vi "Load DC Pins.vi"(8 "error in (no error)":errorcluster, 11 "DCPower in":refnum<class "DCPower.lvclass">) -> (0 "error out":errorcluster, 3 "DCPower out":refnum<class "DCPower.lvclass">)   [LabVIEW 2018, in "DCPower.lvlib" / "DCPower.lvclass"]
uses:
  DCPower.lvclass
  C:/Sequence Automation/Plugins/Measurement Interface.lvlibp/Measurement Interface.lvclass
  DCPower.lvclass/DCPower.ctl
  Write DC Pins.vi
  Plugins/Measurement Interface.lvlibp/Private Methods/Measurement Parameters/Read Measurement Parameters.vi
  Plugins/String Database.lvlibp/String Database.lvclass
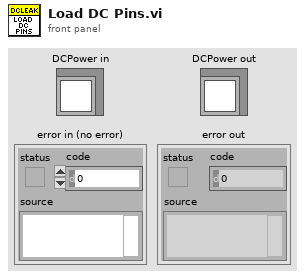
[diagram p1: front panel]
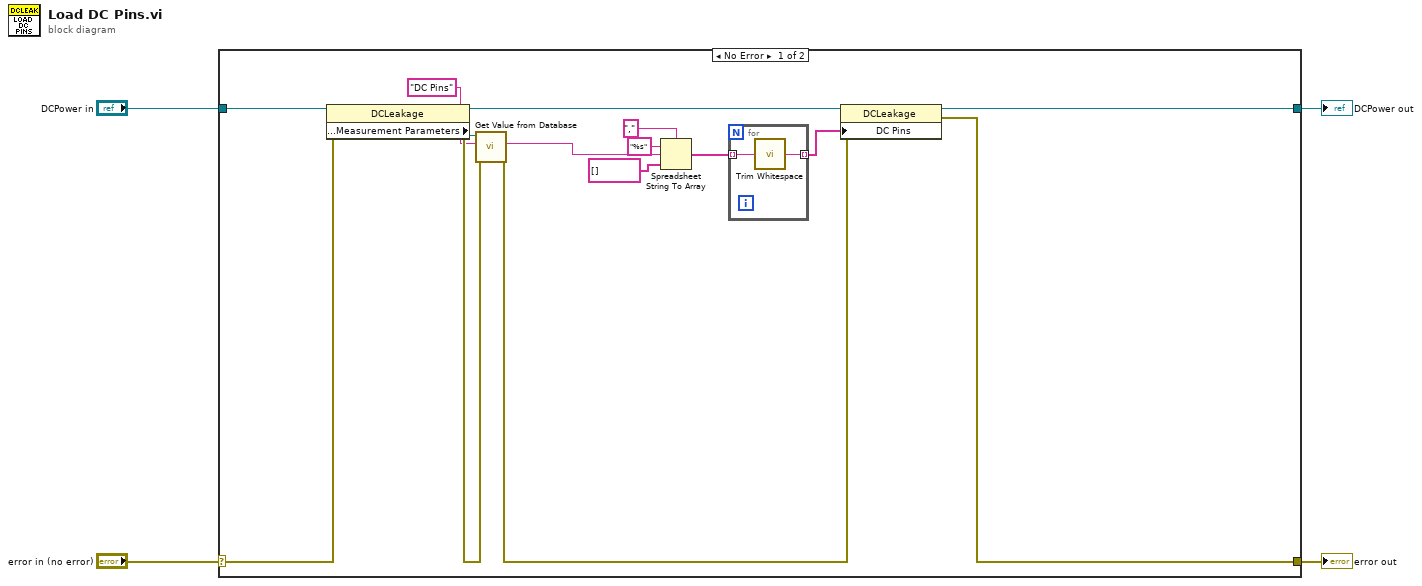
[diagram p0: block diagram]
diagram:
  n1 = case shown="No Error" "error in (no error)" {
    selector: "error in (no error)" -> [w7 w23]
    tunnel: [w6 w23] -> w3
    tunnel: [w5 w22] -> w1
    tunnel: "DCPower in" -> [w8 w22]
    frame No Error {
      n2 = property class="DCLeakage"(reference=w8, error in=w7) -> (reference out=w11:refnum<class "DCPower.lvclass">, error out=w18:errorcluster, "Protected Methods:Measurement Parameters"=w19:refnum<class "String Database.lvclass">)
      n3 = call "Get Value from Database.vi"("error in (no error)"=w18, "Entry Name"="DC Pins", "Message in"=w19) -> ("error out"=w9:errorcluster, "Entry Value"=w14:string)  [unwired: 5 in, 2 out]
      n4 = Spreadsheet String To Array(delimiter (Tab)=",", format string="%s", spreadsheet string=w14, array type (2D Dbl)=string[] []) -> (array=w12:string[])
      n5 = for {
        tunnel: w12 -> [w21] mode=indexing
        tunnel: [w20] -> w10 mode=indexing
        n6 = call <vilib>:"Trim Whitespace.vi"("string"=w21) -> ("trimmed string"=w20:string)  [unwired: 1 in]
      }
      n7 = property class="DCLeakage"(reference=w11, error in=w9, "DC Pins"=w10) -> (reference out=w5:refnum<class "DCPower.lvclass">, error out=w6:errorcluster)
    }
    frame Error {
    }
  }
  "error out" <- w3
  "DCPower out" <- w1
